vi "Addon.Version.Upgrade.vi"(8 "error in (no error)":errorcluster, 11 "Device Item Ref in in":T1 format="%.0x") -> (0 "error out":errorcluster, 3 "Device Item Ref out":T1 format="%.0x")   [LabVIEW 2019, in "Diagnostics Addon Shared.lvlib"]
uses:
  Diagnostics Addon Shared.lvlib
  <vilib>/NI VeriStand/Custom Device API/Custom Device Item Ref.ctl
  Types/Security.Type.ctl
  Types/Settings.Channel.ctl
  <vilib>/NI VeriStand/Custom Device API/Custom Device Channel.ctl
  <vilib>/NI VeriStand/Custom Device API/Custom Device Channel Type.ctl
  NationalInstruments.VeriStand.SystemDefinitionAPI
  Constants.vi
  <vilib>/NI/NI VeriStand Advanced SysDef API/_SubVIs/SysDef.Search.GUID.vi
  <vilib>/NI/NI VeriStand Advanced SysDef API/_SubVIs/SysDef.Property.Get.U32.vi
  <vilib>/NI/NI VeriStand Advanced SysDef API/_SubVIs/SysDef.Property.Get.String.vi
  <vilib>/NI VeriStand/Custom Device API/Custom Device API.lvlib
  <vilib>/NI/NI VeriStand Advanced SysDef API/SysDef API/Advanced System Definition.lvlib
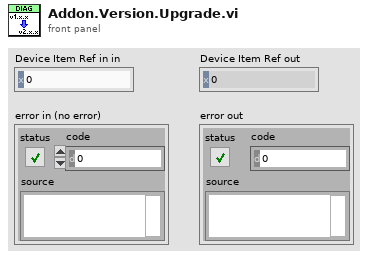
[diagram p1: front panel]
types:
  T1 = typedef "Custom Device API.lvlib/Custom Device Item Ref.ctl" = u64
  T2 = typedef "Diagnostics Addon Shared.lvlib/Security.Type.ctl" = enum16{"None", "SeedKey", "MasterKey"}
  T3 = typedef "Diagnostics Addon Shared.lvlib/Settings.Channel.ctl" = cluster{"Name":string, "Description":string, "Channel":T4}
  T4 = typedef "Custom Device API.lvlib/Custom Device Channel.ctl" = cluster{"Type":T5, "Units":string, "Default Value":dbl, "Faultable":bool, "Scalable":bool}
  T5 = typedef "Custom Device API.lvlib/Custom Device Channel Type.ctl" = enum16{"Input", "Output"}
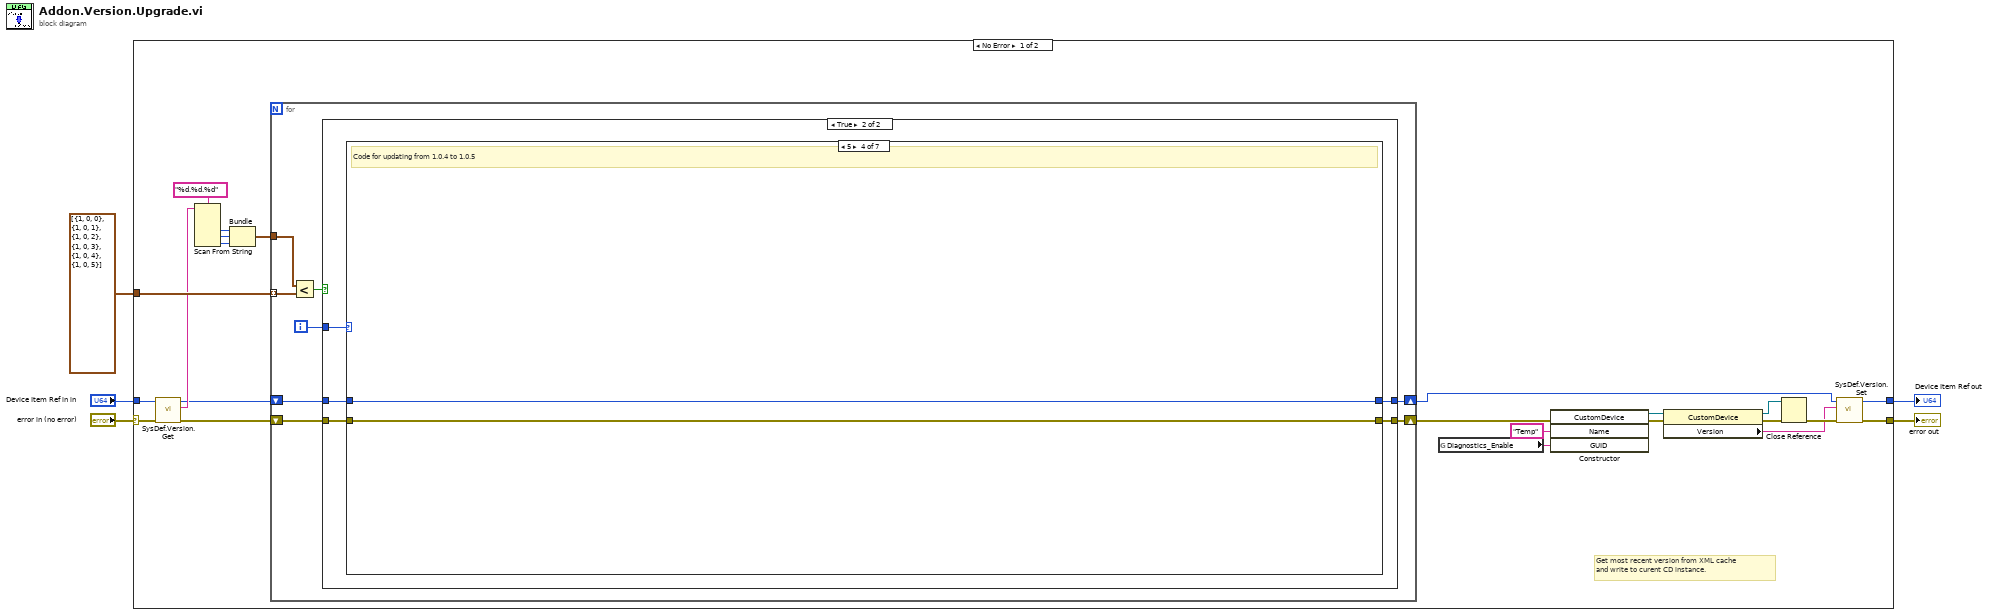
[diagram p0: block diagram]
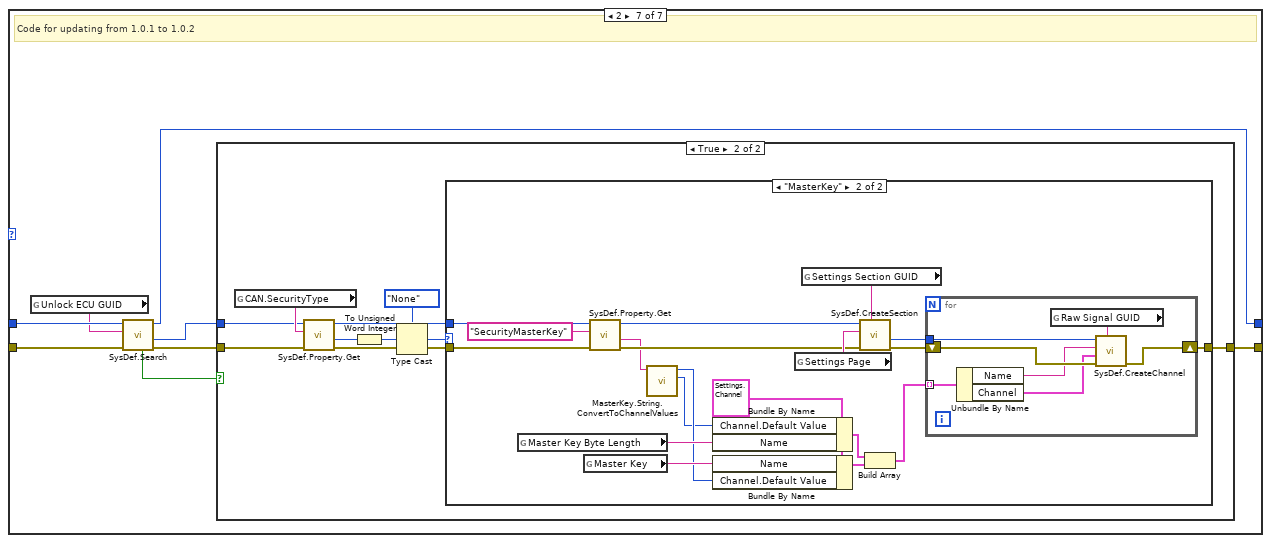
[diagram p8: hidden frame]
diagram:
  n1 = case shown="No Error" "error in (no error)" {
    selector: "error in (no error)" -> [w11 w103]
    tunnel: [w21 w103] -> w4
    tunnel: "Device Item Ref in in" -> [w10 w102]
    tunnel: [w20 w102] -> w5
    tunnel: cluster{i32, i32, i32}[] [{1, 0, 0}, {1, 0, 1}, {1, 0, 2}, {1, 0, 3}, {1, 0, 4}, {1, 0, 5}] -> [w28 _]
    frame No Error {
      # "Get most recent version from XML cache\nand write to curent CD instance."
      n2 = call <vilib>:"SysDef.Version.Get.vi"("error in (no error)"=w11, "nodeID"=w10) -> ("error out"=w7:errorcluster, "Version"=w15:string, "nodeID out"=w6:u64)  [unwired: 7 in]
      n3 = Scan From String(format string="%d.%d.%d", input string=w15) -> (output 1=w13:i32, output 2=w12:i32, output 3=w14:i32)  [unwired: 5 in, 3 out]
      n4 = Bundle(w13, w12, w14) -> (w8:cluster{i32, i32, i32})  [unwired: 1 in]
      n5 = for {
        tunnel: w28 -> [w34] mode=indexing
        shift-right: [w36] -> w19
        shift-left: w7 -> [w30]
        shift-right: [w35] -> w18
        shift-left: w6 -> [w29]
        tunnel: w8 -> [w31]
        i -> [w32]
        n6 = Less?(x=w31, y=w34) -> (x < y?=w33:bool)
        n7 = case shown="True" w33 {
          tunnel: w30 -> [w38 w43]
          tunnel: [w38 w42] -> w36
          tunnel: w29 -> [w37 w39]
          tunnel: [w37 w40] -> w35
          tunnel: w32 -> [_ w41]
          frame False {
          }
          frame True {
            n8 = case shown="5" w41 {
              tunnel: w43 -> [w45 w47 w49 w51 w53 w55 w63]
              tunnel: [w45 w47 w49 w51 w53 w55 w57] -> w42
              tunnel: [w44 w46 w48 w50 w52 w54 w62] -> w40
              tunnel: w39 -> [w44 w46 w48 w50 w52 w54 w61]
              frame Default {
                # "Nothing to update"
              }
              frame 3 {
                # "Code for updating from 1.0.2 to 1.0.3"
              }
              frame 4 {
                # "Code for updating from 1.0.3 to 1.0.4"
              }
              frame 5 {
                # "Code for updating from 1.0.4 to 1.0.5"
              }
              frame 0 {
                # "Initial Onload"
              }
              frame 1 {
                # "Code for updating from 1.0.0 to 1.0.1"
              }
              frame 2 {
                # "Code for updating from 1.0.1 to 1.0.2"
                n9 = global read "Constants.vi" "Unlock ECU GUID"() -> (w56:string)
                n10 = call-poly <vilib>:"SysDef.Search.vi"("error in (no error)"=w63, "GUID"=w56, "nodeID"=w61) -> ("error out"=w59:errorcluster, "Value out"=w58:u64, "nodeID out"=w62:u64, "Found?"=w60:bool)  [unwired: 5 in]
                n11 = case shown="True" w60 {
                  tunnel: w59 -> [w64 w69]
                  tunnel: w58 -> [_ w72]
                  tunnel: [w64 w74] -> w57
                  frame False {
                  }
                  frame True {
                    n12 = global read "Constants.vi" "CAN.SecurityType"() -> (w73:string)
                    n13 = call-poly <vilib>:"SysDef.Property.Get.vi"("error in (no error)"=w69, "Property Name"=w73, "nodeID"=w72) -> ("error out"=w70:errorcluster, "Value out"=w68:u32, "nodeID out"=w71:u64)  [unwired: 5 in, 1 out]
                    n14 = To Unsigned Word Integer(number=w68) -> (unsigned 16bit integer=w67:u16)
                    n15 = Type Cast(type=Security.Type."None" ("Type"), x=w67) -> (*(type *) &x=w65:T2)
                    n16 = case shown="\"MasterKey\"" w65 {
                      tunnel: w70 -> [w75 w88]
                      tunnel: w71 -> [_ w87]
                      tunnel: [w75 w80] -> w74
                      frame Default {
                      }
                      frame "MasterKey" {
                        w90 = T3 {"Name"="Byte Length", "Description"="", "Channel"={"Type"=enum."Input", "Units"="", "Default Value"=0.0, "Faultable"=FALSE, "Scalable"=FALSE}} ("cluster")
                        n17 = global read "Constants.vi" "Master Key Byte Length"() -> (w92:string)
                        n18 = global read "Constants.vi" "Master Key"() -> (w91:string)
                        n19 = call-poly <vilib>:"SysDef.Property.Get.vi"("error in (no error)"=w88, "Property Name"="SecurityMasterKey" ("CAN.SecurityMasterKey"), "nodeID"=w87) -> ("error out"=w82:errorcluster, "Value out"=w79:string, "nodeID out"=w81:u64)  [unwired: 5 in, 1 out]
                        n20 = call "MasterKey.String.ConvertToChannelValues.vi"("Master Key"=w79) -> ("Length"=w76:i32, "Value"=w77:u64)  [unwired: 9 in]
                        n21 = Bundle By Name(cluster=w90, "Channel.Default Value"=w76, "Name"=w92) -> (w93:T3)
                        n22 = Bundle By Name(cluster=w90, "Name"=w91, "Channel.Default Value"=w77) -> (w94:T3)
                        n23 = global read "Constants.vi" "Settings Page"() -> (w86:string)
                        n24 = global read "Constants.vi" "Settings Section GUID"() -> (w85:string)
                        n25 = call <vilib>:"SysDef.CreateSection.vi"("GUID"=w85, "error in (no error)"=w82, "Name"=w86, "nodeID"=w81) -> ("error out"=w83:errorcluster, "New NodeID"=w84:u64)  [unwired: 4 in, 2 out]
                        n26 = Build Array(w93, w94) -> (w78:T3[])
                        n27 = for {
                          tunnel: w84 -> [w99]
                          shift-right: [w98] -> w80
                          shift-left: w83 -> [w100]
                          tunnel: w78 -> [w95] mode=indexing
                          n28 = Unbundle By Name(w95) -> ("Name"=w97:string, "Channel"=w96:T4)
                          n29 = global read "Constants.vi" "Raw Signal GUID"() -> (w101:string)
                          n30 = call <vilib>:"SysDef.CreateChannel.vi"("GUID"=w101, "error in (no error)"=w100, "Channel"=w96, "Name"=w97, "nodeID"=w99) -> ("error out"=w98:errorcluster)  [unwired: 3 in, 3 out]
                        }
                      }
                    }
                  }
                }
              }
            }
          }
        }
      }
      n31 = global read "Constants.vi" "Diagnostics_Enable"() -> (w16:string)
      n32 = constructor class="CustomDevice"(error in=w19, "Name"="Temp", "GUID"=w16) -> (reference out=w27:refnum<k24>, error out=w26:errorcluster)  [unwired: 2 in, 3 out]
      n33 = property class="CustomDevice"(reference=w27, error in=w26) -> (reference out=w24:refnum<k24>, error out=w25:errorcluster, "Version"=w22:string)
      n34 = Close Reference(reference=w24, error in (no error)=w25) -> (error out=w23:errorcluster)
      n35 = call <vilib>:"SysDef.Version.Set.vi"("error in (no error)"=w23, "Version"=w22, "nodeID"=w18) -> ("error out"=w21:errorcluster, "nodeID out"=w20:u64)  [unwired: 7 in]
    }
    frame Error {
    }
  }
  "Device Item Ref out" <- w5
  "error out" <- w4
